vi "Check for Reboot Loop.vi"() -> (2 "Start in Safe Mode?":bool)   [LabVIEW 2022 SP3]
uses:
  Globals/Global - Configuration Options.vi
  <vilib>/Utility/file.llb/Read From Spreadsheet File (string).vi
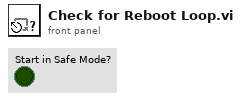
[diagram p1: front panel]
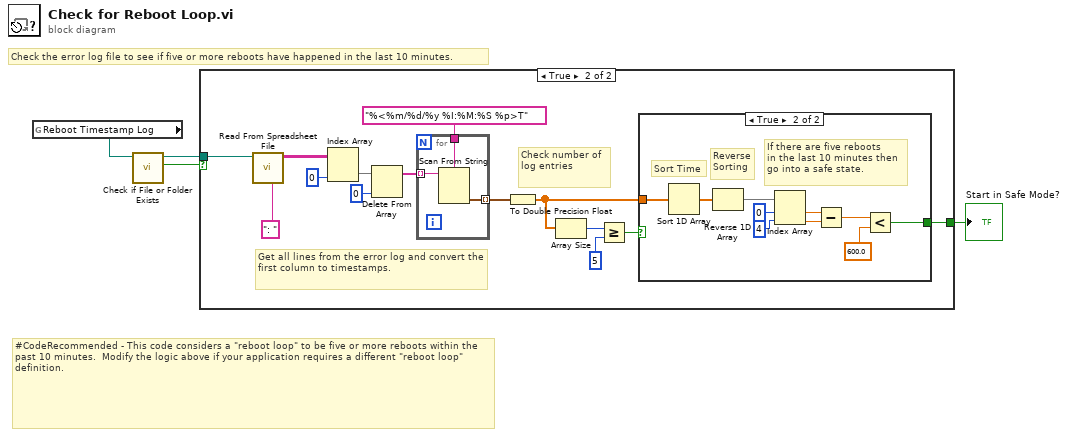
[diagram p0: block diagram]
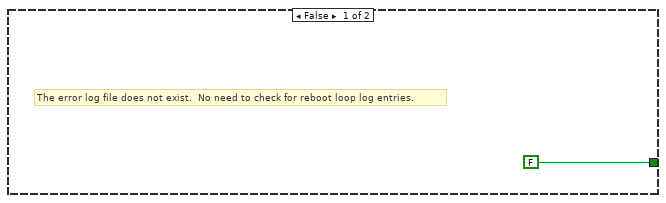
[diagram p2: hidden frame]
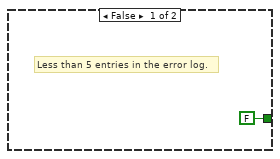
[diagram p3: hidden frame]
diagram:
  # "#CodeRecommended - This code considers a \"reboot loop\" to be five or more reboots within the past 10 minutes.  Modify the logic above if your application requires a different \"reboot loop\" definition."
  # "Check the error log file to see if five or more reboots have happened in the last 10 minutes."
  n1 = global read "Global - Configuration Options.vi" "Reboot Timestamp Log"() -> (w1:path)
  n2 = call <vilib>:"Check if File or Folder Exists.vi"("path"=w1) -> ("file or folder exists?"=w4:bool, "dup path"=w3:path)  [unwired: 8 in, 1 out]
  n3 = case shown="True" w4 {
    tunnel: w3 -> [_ w19]
    tunnel: [FALSE w14] -> w2
    frame False {
      # "The error log file does not exist.  No need to check for reboot loop log entries."
    }
    frame True {
      # "Check number of log entries"
      # "Get all lines from the error log and convert the first column to timestamps."
      n4 = call-poly <vilib>:"Read From Spreadsheet File.vi"("delimiter (\\t)"=": " ("delimiter (\\t)"), "file path (dialog if empty)"=w19) -> ("all rows"=w18:string[][])  [unwired: 5 in, 4 out]
      n5 = Index Array(array=w18, index (col)=0 ("disabled index (col)")) -> (element=w8:string[])  [unwired: 1 in]
      n6 = Delete From Array(array=w8, index=0) -> (array with subset deleted=w7:string[])  [unwired: 1 in, 1 out]
      n7 = for {
        tunnel: w7 -> [w33] mode=indexing
        tunnel: "%<%m/%d/%y %I:%M:%S %p>T" -> [w32]
        tunnel: [w31] -> w15 mode=indexing
        n8 = Scan From String(format string=w32, input string=w33) -> (output 1=w31:timestamp)  [unwired: 3 in, 3 out]
      }
      n9 = To Double Precision Float(number=w15) -> (double precision float=w13:dbl[])
      n10 = Array Size(array=w13) -> (size(s)=w12:i32)
      n11 = Greater Or Equal?(x=w12, y=5) -> (x >= y?=w10:bool)
      n12 = case shown="True" w10 {
        tunnel: [FALSE w22] -> w14
        tunnel: w13 -> [_ w21]
        frame False {
          # "Less than 5 entries in the error log."
        }
        frame True {
          # "If there are five reboots\nin the last 10 minutes then\ngo into a safe state."
          # "Reverse\nSorting"
          # "Sort Time"
          n13 = Sort 1D Array(array=w21) -> (sorted array=w30:dbl[])
          n14 = Reverse 1D Array(array=w30) -> (reversed array=w29:dbl[])
          n15 = Index Array(array=w29, index #1=0 ("index"), index #2=4 ("index")) -> (element #1=w26:dbl, element #2=w25:dbl)
          n16 = Subtract(x=w26, y=w25) -> (x-y=w24:dbl)
          n17 = Less?(x=w24, y=600.0) -> (x < y?=w22:bool)
        }
      }
    }
  }
  "Start in Safe Mode?" <- w2
